vi "Grab Communications Properties.vi"(0 "Communications Setup":T1={"IP Address"="192.168.0.222", "VISA Resource Name"="GPIB0::4::INSTR", "Scheme"=0} {"Scheme" items=["Ethernet Auto", "GPIB Auto", "Ethernet Manual", "GPIB & RS232 Manual"]}) -> (1 "Use VISA":bool, 2 "VISA Resource Name out":refnum<visa-resource-name>="GPIB0::4::INSTR", 3 "IP Address":string="192.168.0.222")   [LabVIEW 2010]
uses:
  Communications Setup.ctl
panel:
  in  "error in (no error) 2":errorcluster
  in  "error in (no error)":errorcluster
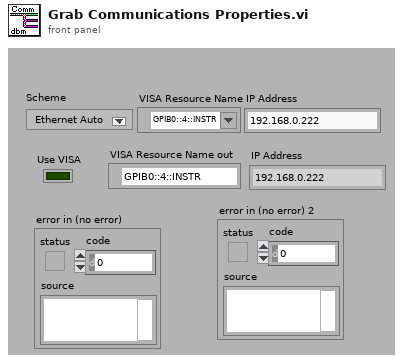
[diagram p1: front panel]
types:
  T1 = typedef "Communications Setup.ctl" = cluster{"IP Address":string, "VISA Resource Name":refnum<visa-resource-name>, "Scheme":u16}
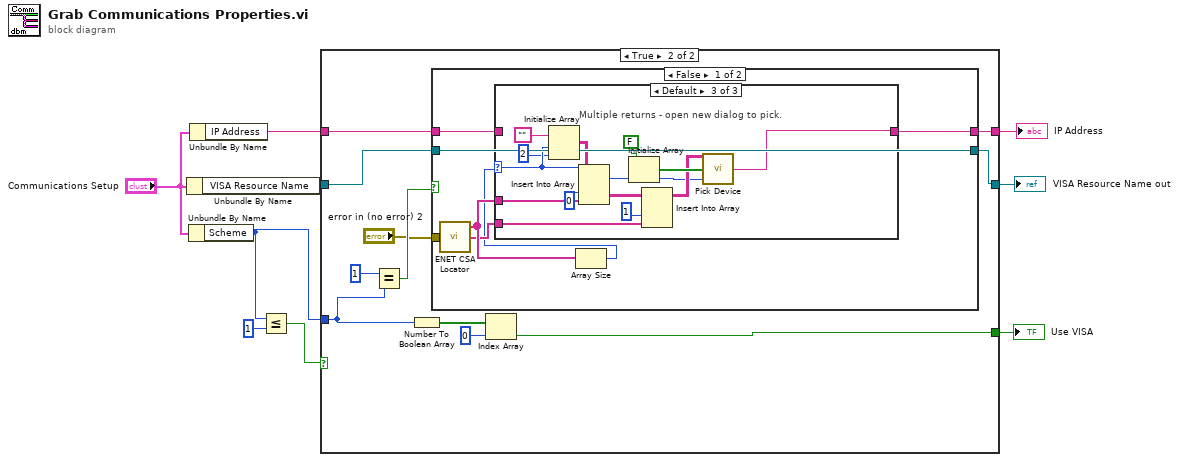
[diagram p0: block diagram]
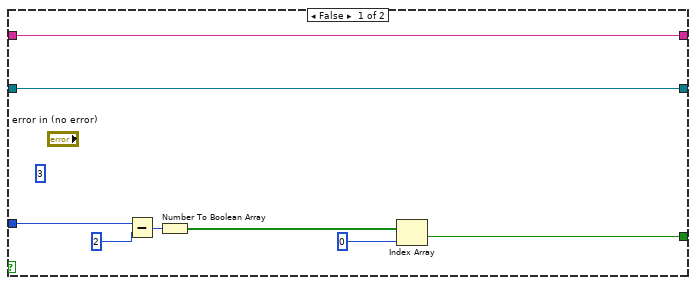
[diagram p2: hidden frame]
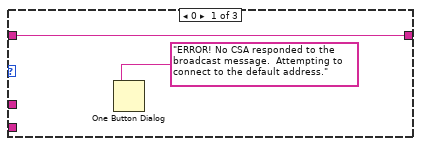
[diagram p3: hidden frame]
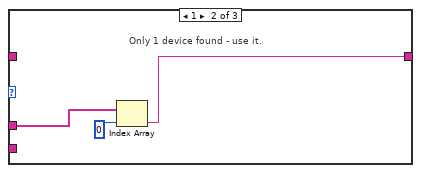
[diagram p4: hidden frame]
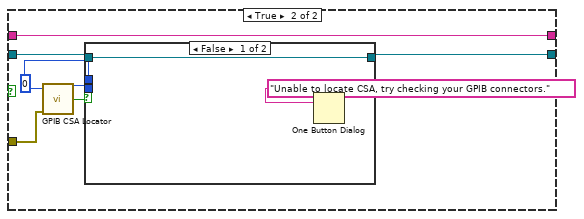
[diagram p5: hidden frame]
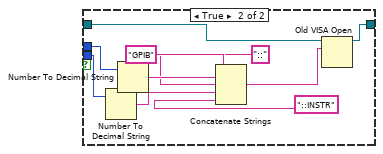
[diagram p6: hidden frame]
diagram:
  n1 = Unbundle By Name("Communications Setup") -> ("VISA Resource Name"=w2:refnum<visa-resource-name>)
  n2 = Unbundle By Name("Communications Setup") -> ("Scheme"=w8:u16)
  n3 = Unbundle By Name("Communications Setup") -> ("IP Address"=w4:string)
  n4 = Less Or Equal?(x=w8, y=1) -> (x <= y?=w6:bool)
  n5 = case shown="True" w6 {
    tunnel: w8 -> [w13 w23]
    tunnel: [w15 w26] -> w5
    tunnel: [w14 w18] -> w1
    tunnel: w2 -> [w14 w20]
    tunnel: [w10 w19] -> w3
    tunnel: w4 -> [w10 w21]
    frame False {
      (unwired) 3
      n6 = Subtract(x=w13, y=2) -> (x-y=w11:i32)
      n7 = Number To Boolean Array(number=w11) -> (Boolean array=w16:bool[])
      n8 = Index Array(array=w16, index=0) -> (element=w15:bool)
    }
    frame True {
      n9 = Equal?(x=1, y=w23) -> (x = y?=w25:bool)
      n10 = Number To Boolean Array(number=w23) -> (Boolean array=w27:bool[])
      n11 = case shown="False" w25 {
        tunnel: [w35 w59] -> w18
        tunnel: w20 -> [w35 w58]
        tunnel: [w34 w55] -> w19
        tunnel: w21 -> [w33 w55]
        tunnel: "error in (no error) 2" -> [w32 w54]
        frame False {
          n12 = call "ENET CSA Locator.vi"("error in (no error)"=w32) -> ("IP Array"=w31:string[], "Data Return Array"=w30:string[])  [unwired: 1 out]
          n13 = Array Size(array=w31) -> (size(s)=w29:i32)
          n14 = case shown="Default" w29 {
            selector: w29 -> [_ _ w42]
            tunnel: [w36 w38 w53] -> w34
            tunnel: w33 -> [w36 _ _]
            tunnel: w31 -> [_ w40 w44]
            tunnel: w30 -> [_ _ w50]
            frame 0 {
              n15 = One Button Dialog(message="ERROR! No CSA responded to the broadcast message.  Attempting to connect to the default address.") -> ()  [unwired: 1 in, 1 out]
            }
            frame 1 {
              # "Only 1 device found - use it."
              n16 = Index Array(array=w40, index=0) -> (element=w38:string)
            }
            frame Default {
              # "Multiple returns - open new dialog to pick."
              n17 = Initialize Array("", w42, 2) -> (w48:string[][])
              n18 = Insert Into Array(array=w48, index (col)=0, new element=w44) -> (w47:string[][])  [unwired: 1 in]
              n19 = Initialize Array(FALSE, w42) -> (w52:bool[])
              n20 = Insert Into Array(array=w47, index (col)=1, new element=w50) -> (w46:string[][])  [unwired: 1 in]
              n21 = call "Pick Device.vi"("Max Devices"=w42, "Device Selected"=w52, "Available Devices:"=w46) -> ("Return Address"=w53:string)
            }
          }
        }
        frame True {
          w57 = 0
          n22 = call "GPIB CSA Locator.vi"("GPIB Bus"=w57, "error in (no error)"=w54) -> ("CSA Address"=w56:i32, "Found Address"=w60:bool)  [unwired: 1 out]
          n23 = case shown="False" w60 {
            tunnel: [w61 w64] -> w59
            tunnel: w58 -> [w61 w65]
            tunnel: w57 -> [_ w70]
            tunnel: w56 -> [_ w69]
            frame False {
              n24 = One Button Dialog(message="Unable to locate CSA, try checking your GPIB connectors.") -> ()  [unwired: 1 in, 1 out]
            }
            frame True {
              n25 = Number To Decimal String(number=w69) -> (decimal integer string=w67:string)  [unwired: 1 in]
              n26 = Number To Decimal String(number=w70) -> (decimal integer string=w71:string)  [unwired: 1 in]
              n27 = Concatenate Strings("GPIB", w71, "::", w67, "::INSTR") -> (w63:string)
              n28 = Old VISA Open(10:w63, 11:w65) -> (3:w64:refnum<visa-resource-name>)  [unwired: 3 in, 1 out]
            }
          }
        }
      }
      n29 = Index Array(array=w27, index=0) -> (element=w26:bool)
    }
  }
  "VISA Resource Name out" <- w1
  "IP Address" <- w3
  "Use VISA" <- w5
